vi "Generate_WayPoints_Hopping_SelfReference.vi"(11 "Input Cluster":T2={"Scan Rate (um/s)"=15.0, "X Start"=15.0, "X End"=15.0, "Y Start"=15.0, "Y End"=15.0, " Z Start"=15.0, "HoppingDistance"=1.0, "V"=15.0, "Z End"=15.0, "Approach Rate Hopping (um/s)"=15.0, "Retract Rate (um/s)"=15.0, "V 2"=15.0, "Approach Rate (um/s)"=15.0}) -> (0 "output cluster":T1)   [LabVIEW 2023]
uses:
  TypeDefs/WayPointCluster.ctl
  User_Vi/Settings.vi
panel:
  in  "WayPointCluster":T1
  out "Y  P":dbl
  out "X  P":dbl
  out "HoppingDistanceX":dbl
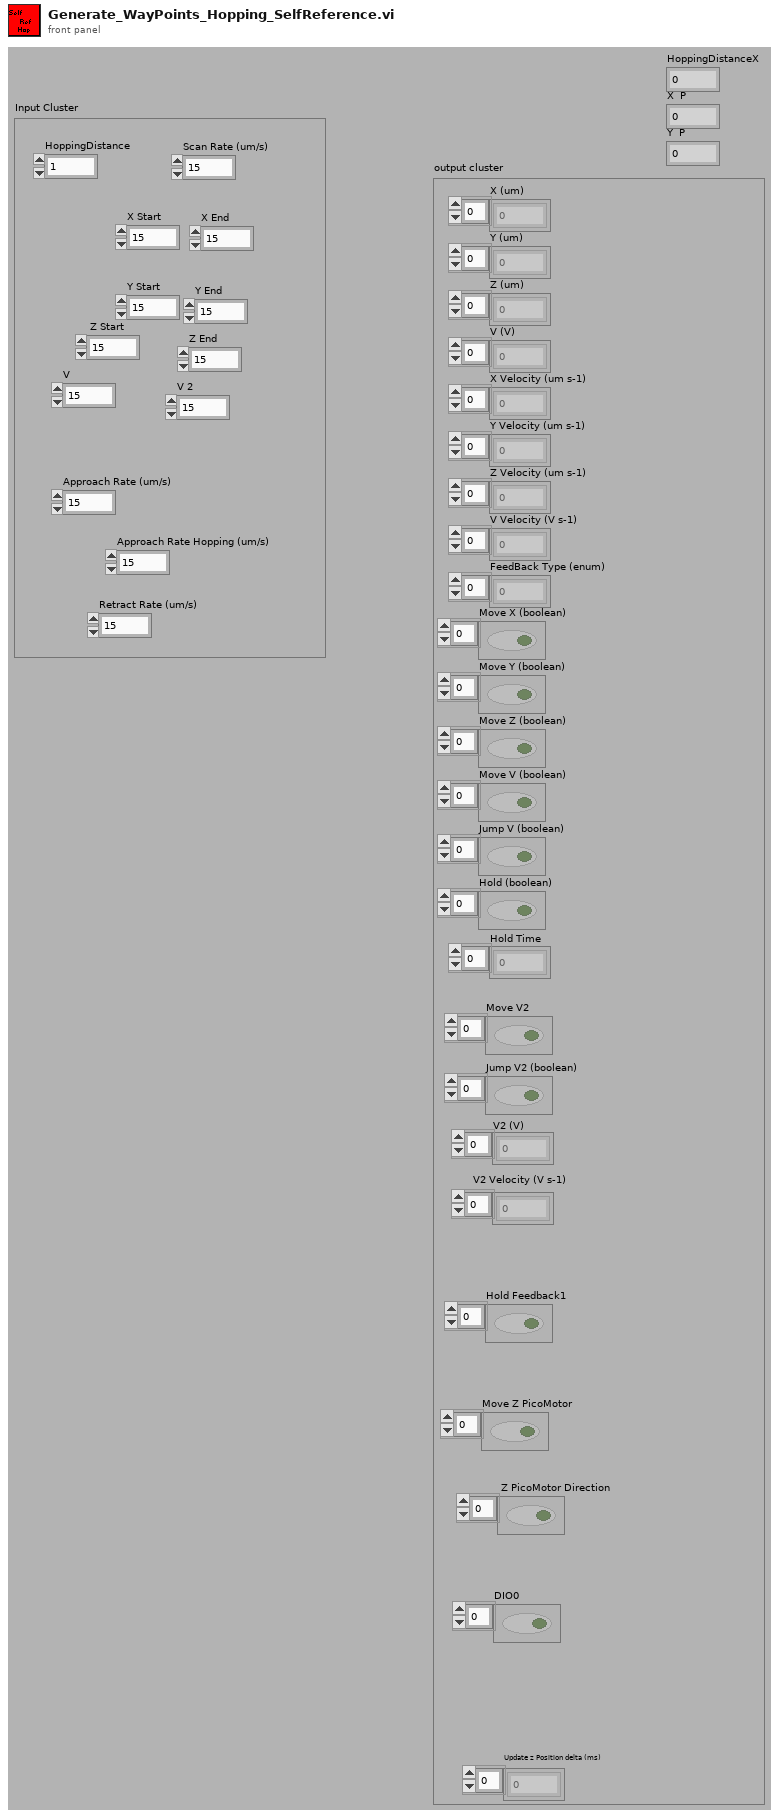
[diagram p1: front panel]
types:
  T1 = typedef "WayPointCluster.ctl" = cluster{"X (um)":dbl[], "Y (um)":dbl[], "Z (um)":dbl[], "V (V)":dbl[], "X Velocity (um s-1)":dbl[], "Y Velocity (um s-1)":dbl[], "Z Velocity (um s-1)":dbl[], "V Velocity (V s-1)":dbl[], "FeedBack Type (enum)":u16[], "Move X (boolean)":bool[], "Move Y (boolean)":bool[], "Move Z (boolean)":bool[], "Move V (boolean)":bool[], "Jump V (boolean)":bool[], "Hold (boolean)":bool[], "Hold Time":u32[], "V2 (V)":dbl[], "Move V2":bool[], "V2 Velocity (V s-1)":dbl[], "Jump V2 (boolean)":bool[], "Update z Position delta (ms)":i16[], "Hold Feedback1":bool[], "Move Z PicoMotor":bool[], " Z PicoMotor Direction":bool[], "DIO0":bool[]}
  T2 = cluster{"Scan Rate (um/s)":dbl, "X Start":dbl, "X End":dbl, "Y Start":dbl, "Y End":dbl, " Z Start":dbl, "HoppingDistance":dbl, "V":dbl, "Z End":dbl, "Approach Rate Hopping (um/s)":dbl, "Retract Rate (um/s)":dbl, "V 2":dbl, "Approach Rate (um/s)":dbl}
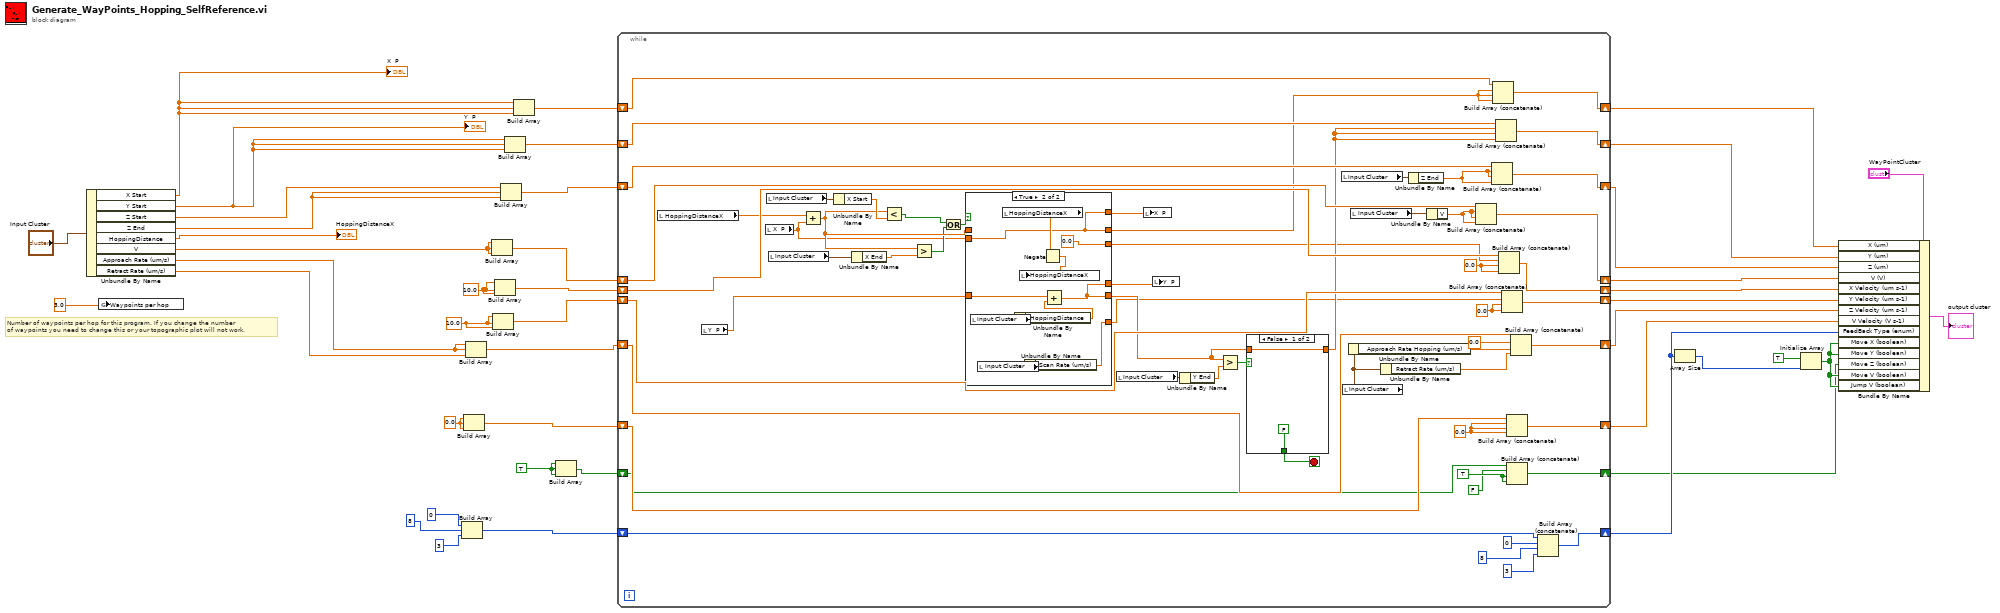
[diagram p0: block diagram]
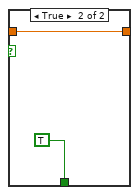
[diagram p2: hidden frame]
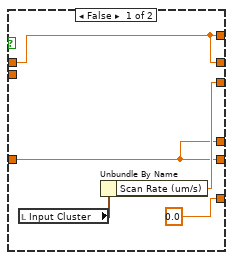
[diagram p3: hidden frame]
diagram:
  w2 = TRUE
  w12 = 10.0 ("element")
  w11 = 10.0 ("element")
  w9 = 0.0 ("element")
  # "Number of waypoints per hop for this program. If you change the number\nof waypoints you need to change this or your topographic plot will not work."
  n1 = Unbundle By Name("Input Cluster") -> ("X Start"=w24:dbl, "Y Start"=w18:dbl, "Z Start"=w17:dbl, "Z End"=w14:dbl, "HoppingDistance"=→"HoppingDistanceX":dbl, "V"=w15:dbl, "Approach Rate (um/s)"=w10:dbl, "Retract Rate (um/s)"=w23:dbl)
  "X  P" <- w24
  "Y  P" <- w18
  n2 = global write "Settings.vi" "Waypoints per hop"(3.0) -> ()
  n3 = Build Array(u16 0 ("element"), u16 8 ("element"), u16 3 ("element")) -> (w25:u16[])
  n4 = Build Array(w9, w9, w9) -> (w27:dbl[])
  n5 = Build Array(w10, w10, w23) -> (w29:dbl[])
  n6 = Build Array(w15, w15, w15) -> (w34:dbl[])
  n7 = Build Array(w11, w11, w11) -> (w31:dbl[])
  n8 = Build Array(w12, w12, w12) -> (w32:dbl[])
  n9 = Build Array(w17, w14, w14) -> (w36:dbl[])
  n10 = Build Array(w18, w18, w18) -> (w37:dbl[])
  n11 = Build Array(w24, w24, w24) -> (w39:dbl[])
  n12 = Build Array(w2, w2, w2) -> (w3:bool[])
  n13 = while {
    shift-right: [w97] -> w38
    shift-left: w39 -> [w98]
    shift-right: [w89] -> w19
    shift-left: w37 -> [w79]
    shift-right: [w88] -> w35
    shift-left: w36 -> [w96]
    shift-right: [w87] -> w33
    shift-left: w34 -> [w95]
    shift-right: [w86] -> w20
    shift-left: w32 -> [w94]
    shift-right: [w85] -> w30
    shift-left: w31 -> [w93]
    shift-right: [w84] -> w28
    shift-left: w29 -> [w92]
    shift-right: [w83] -> w26
    shift-left: w27 -> [w91]
    shift-right: [w82] -> w16
    shift-left: w25 -> [w90]
    shift-right: [w44] -> w4
    shift-left: w3 -> [w43]
    stop <- w69 stop-if-true
    w46 = TRUE
    w51 = 0.0 ("element")
    w52 = 0.0 ("element")
    w65 = 0.0 ("element")
    n14 = local read "HoppingDistanceX"() -> (w48:dbl)
    n15 = local read "Y  P"() -> (w63:dbl)
    n16 = local read "X  P"() -> (w49:dbl)
    n17 = local read "Input Cluster"() -> (w100:T2)
    n18 = local read "Input Cluster"() -> (w99:T2)
    n19 = Add(x=w48, y=w49) -> (x+y=w75:dbl)
    n20 = Unbundle By Name(w100) -> ("X Start"=w78:dbl)
    n21 = Unbundle By Name(w99) -> ("X End"=w76:dbl)
    n22 = Less?(x=w75, y=w78) -> (x < y?=w77:bool)
    n23 = Greater?(x=w75, y=w76) -> (0:w74:bool)
    n24 = Or(x=w77, y=w74) -> (x .or. y?=w73:bool)
    n25 = case shown="True" w73 {
      tunnel: w75 -> [w105 _]
      tunnel: [w105 w111] -> w62
      tunnel: w49 -> [_ w111]
      tunnel: w63 -> [w106 w112]
      tunnel: [w106 w110] -> w61
      tunnel: [w108 0.0] -> w53
      tunnel: [0.0 w113] -> w50
      tunnel: [w106 w110] -> w60
      tunnel: [w105 w111] -> w59
      frame False {
        n26 = local read "Input Cluster"() -> (w109:T2)
        n27 = Unbundle By Name(w109) -> ("Scan Rate (um/s)"=w108:dbl)
      }
      frame True {
        n28 = local read "Input Cluster"() -> (w117:T2)
        n29 = local read "Input Cluster"() -> (w115:T2)
        n30 = local read "HoppingDistanceX"() -> (w119:dbl)
        n31 = Unbundle By Name(w117) -> ("HoppingDistance"=w116:dbl)
        n32 = Unbundle By Name(w115) -> ("Scan Rate (um/s)"=w113:dbl)
        n33 = Negate(x=w119) -> (-x=w118:dbl)
        n34 = local write "HoppingDistanceX"(w118) -> ()
        n35 = Add(x=w112, y=w116) -> (x+y=w110:dbl)
      }
    }
    n36 = local read "Input Cluster"() -> (w72:T2)
    n37 = local write "X  P"(w59) -> ()
    n38 = local write "Y  P"(w60) -> ()
    n39 = Unbundle By Name(w72) -> ("Y End"=w71:dbl)
    n40 = Greater?(x=w61, y=w71) -> (0:w70:bool)
    n41 = case shown="False" w70 {
      tunnel: w61 -> [w102 w104]
      tunnel: [w102 w104] -> w68
      tunnel: [FALSE TRUE] -> w69
      frame False {
      }
      frame True {
      }
    }
    n42 = local read "Input Cluster"() -> (w81:T2)
    n43 = local read "Input Cluster"() -> (w64:T2)
    n44 = Unbundle By Name(w64) -> ("Approach Rate Hopping (um/s)"=w55:dbl)
    n45 = local read "Input Cluster"() -> (w80:T2)
    n46 = Unbundle By Name(w64) -> ("Retract Rate (um/s)"=w54:dbl)
    n47 = Unbundle By Name(w81) -> ("Z End"=w67:dbl)
    n48 = Unbundle By Name(w80) -> ("V"=w66:dbl)
    n49 = Build Array (concatenate)(w95, w66, w66, w66) -> (w87:dbl[])
    n50 = Build Array (concatenate)(w96, w67, w67, w67) -> (w88:dbl[])
    n51 = Build Array (concatenate)(w98, w62, w62, w62) -> (w97:dbl[])
    n52 = Build Array (concatenate)(w79, w68, w68, w68) -> (w89:dbl[])
    n53 = Build Array (concatenate)(w94, w53, w52, w52) -> (w86:dbl[])
    n54 = Build Array (concatenate)(w93, w50, w51, w51) -> (w85:dbl[])
    n55 = Build Array (concatenate)(w91, w65, w65, w65) -> (w83:dbl[])
    n56 = Build Array (concatenate)(w43, FALSE, w46, w46) -> (w44:bool[])
    n57 = Build Array (concatenate)(w92, 0.0 ("element"), w55, w54) -> (w84:dbl[])
    n58 = Build Array (concatenate)(w90, u16 0 ("element"), u16 8 ("element"), u16 3 ("element")) -> (w82:u16[])
  }
  n59 = Array Size(array=w16) -> (size(s)=w21:i32)
  n60 = Initialize Array(TRUE, w21) -> (w40:bool[])
  n61 = Bundle By Name(cluster="WayPointCluster", "X (um)"=w38, "Y (um)"=w19, "Z (um)"=w35, "V (V)"=w33, "X Velocity (um s-1)"=w20, "Y Velocity (um s-1)"=w30, "Z Velocity (um s-1)"=w28, "V Velocity (V s-1)"=w26, "FeedBack Type (enum)"=w16, "Move X (boolean)"=w40, "Move Y (boolean)"=w40, "Move Z (boolean)"=w4, "Move V (boolean)"=w40, "Jump V (boolean)"=w40) -> (→"output cluster":T1)
